vi "ClusterEscala.vi"() -> ()   [LabVIEW 2020]
panel:
  out "Cluster 2":T1 {"Gauge" scale=0.0..100.0; "Tank" scale=0.0..100.0; "Thermometer" scale=0.0..100.0}
  in  "Cluster":T2
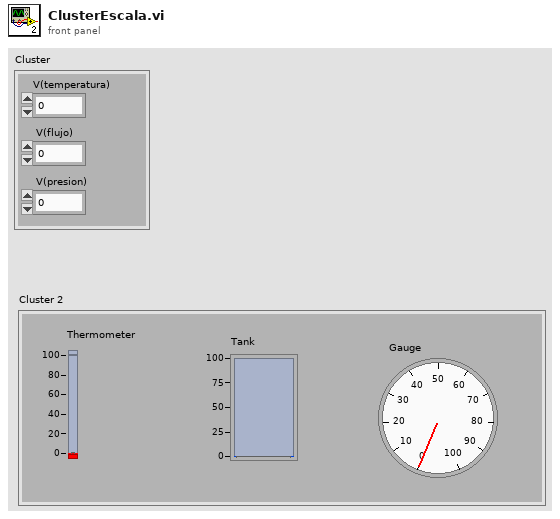
[diagram p1: front panel]
types:
  T1 = cluster{"Thermometer":dbl, "Tank":dbl, "Gauge":dbl}
  T2 = cluster{" V(flujo)":dbl, " V(presion)":dbl, "V(temperatura)":dbl}
  T3 = cluster{"°C/V":i32, "(I/seg)/V":i32, "(N/m^2)/V":i32}
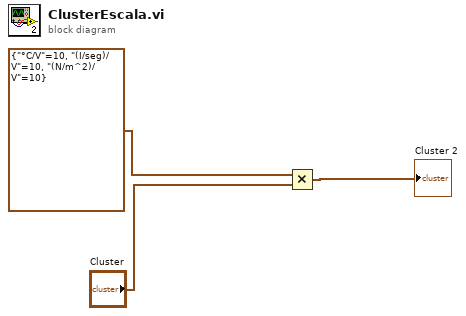
[diagram p0: block diagram]
diagram:
  n1 = Multiply(x=T3 {"°C/V"=10, "(I/seg)/V"=10, "(N/m^2)/V"=10}, y="Cluster") -> (x*y=→"Cluster 2":cluster{dbl, dbl, dbl})
